vi "NT Process Queued Updates.vi"(9 "Bound Names":string[](array[string]), 11 "handles":cluster{"poller":u32, "topicListener":u32}) -> (3 "Updates":variant[](array[variant]))   [LabVIEW 2025]
uses:
  59b6e50f-ea3d-427c-8cdf-50e68eee575c.vi
  55de3b79-44e1-4c34-8f24-7fb90773489e.vi
  6bfa8e3a-c1d4-42b7-80f0-8f7f4c5a93ba.vi
  b6a8a16d-f334-414e-a614-8fde72f469f3.vi
  <vilib>/Rock Robotics/Network Tables/NT Globals.vi
  <vilib>/Comparison/Equal/Equal Functor/Equal Functor.lvclass
  FRC_NetworkTablesLV.dll
  ntcoreffi.dll
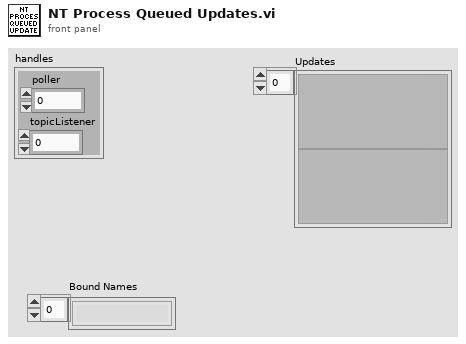
[diagram p1: front panel]
types:
  T1 = cluster{dbl, sgl, i64, string, bool[], dbl[], sgl[], i64[], string[], bool}
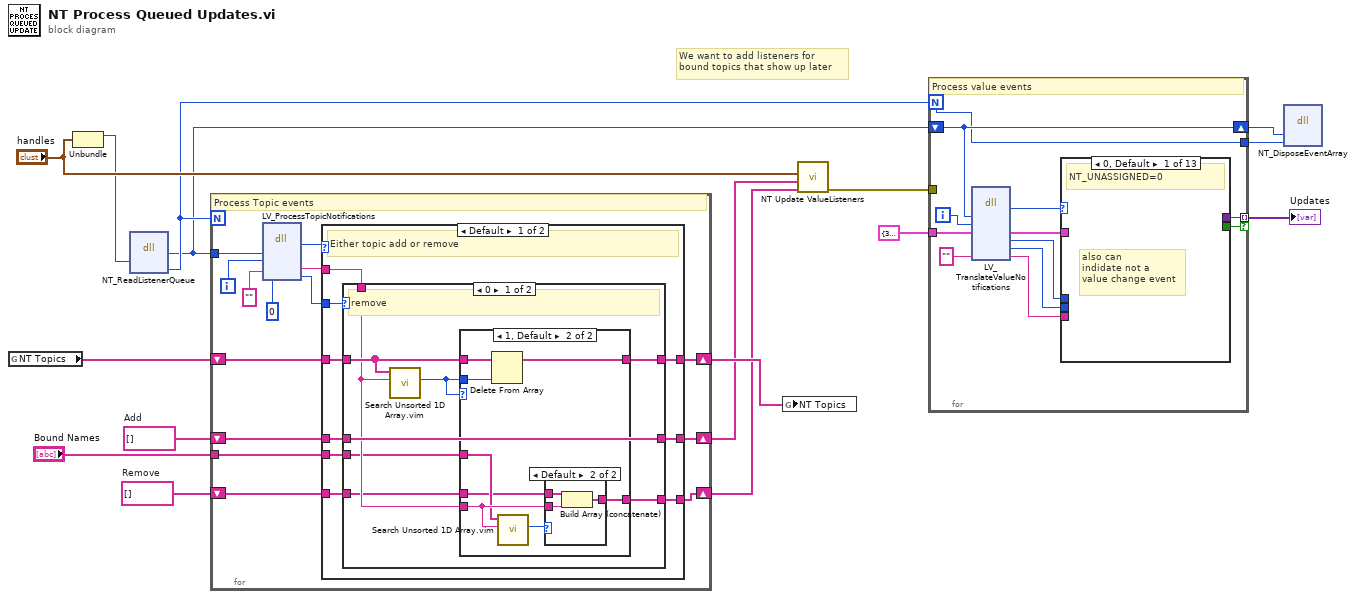
[diagram p0: block diagram]
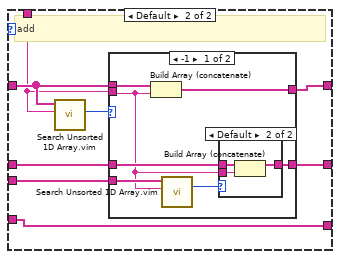
[diagram p4: hidden frame]
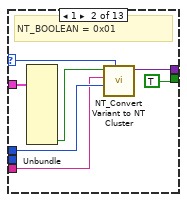
[diagram p8: hidden frame]
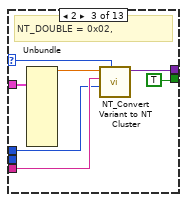
[diagram p9: hidden frame]
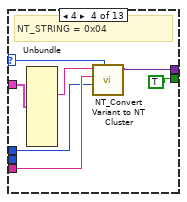
[diagram p10: hidden frame]
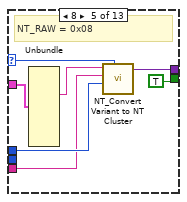
[diagram p11: hidden frame]
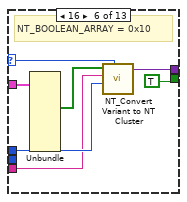
[diagram p12: hidden frame]
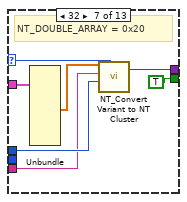
[diagram p13: hidden frame]
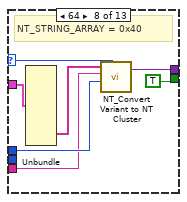
[diagram p14: hidden frame]
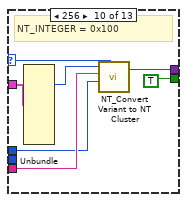
[diagram p16: hidden frame]
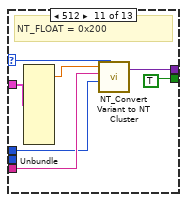
[diagram p17: hidden frame]
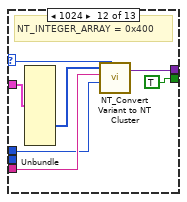
[diagram p18: hidden frame]
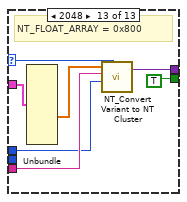
[diagram p19: hidden frame]
diagram:
  w3 = string[] []  # Remove
  w10 = string[] []  # Add
  # "We want to add listeners for\nbound topics that show up later"
  n1 = global read "NT Globals.vi" "NT Topics"() -> (w11:string[])
  n2 = Unbundle("handles") -> ("poller"=w1:u32)  [unwired: 1 out]
  n3 = dll-call lib="ntcoreffi.*" fn="NT_ReadListenerQueue"("poller"=w1) -> ("topicNotif"=w5:u64, "count"=w6:u64)  [unwired: 5 in, 2 out]
  n4 = for {
    N: w6 -> [_]
    tunnel: w5 -> [w30]
    shift-right: [w26] -> w12
    shift-left: w11 -> [w27]
    shift-right: [w24] -> w8
    shift-left: w10 -> [w25]
    tunnel: "Bound Names" -> [w23]
    shift-right: [w17] -> w2
    shift-left: w3 -> [w18]
    i -> [w29]
    # "Process Topic events"
    n5 = dll-call lib="FRC_NetworkTablesLV.*" fn="LV_ProcessTopicNotifications"("topicNotifierArray"=w30, "index"=w29, "name"="", "add"=0) -> ("type"=w21:i32, "name"=w22:string, "add"=w20:i32)  [unwired: 5 in, 2 out]
    n6 = case shown="Default" w21 {
      tunnel: w27 -> [w38 w85]
      tunnel: [w39 w85] -> w26
      tunnel: w25 -> [w37 w84]
      tunnel: [w36 w84] -> w24
      tunnel: w23 -> [w35 _]
      tunnel: w22 -> [w34 _]
      tunnel: w20 -> [w33 _]
      tunnel: w18 -> [w32 w83]
      tunnel: [w31 w83] -> w17
      frame Default {
        # "Either topic add or remove"
        n7 = case shown="0" w33 {
          tunnel: [w46 w69] -> w39
          tunnel: w38 -> [w47 w68]
          tunnel: w37 -> [w44 w66]
          tunnel: [w44 w65] -> w36
          tunnel: w35 -> [w40 w64]
          tunnel: w34 -> [w43 w63]
          tunnel: w32 -> [w42 w62]
          tunnel: [w41 w62] -> w31
          frame 0 {
            # "remove"
            n8 = call "Search Unsorted 1D Array.vim"("element"=w43, "unsorted 1D array"=w47) -> ("index of element"=w45:i32)  [unwired: 9 in]
            n9 = case shown="1, Default" w45 {
              tunnel: w47 -> [w49 w57]
              tunnel: [w49 w56] -> w46
              tunnel: w45 -> [_ w55]
              tunnel: w43 -> [_ w52]
              tunnel: w42 -> [w48 w50]
              tunnel: [w48 w53] -> w41
              tunnel: w40 -> [_ w51]
              frame -1 {
              }
              frame 1, Default {
                n10 = Delete From Array(array=w57, index=w55) -> (array with subset deleted=w56:string[])  [unwired: 1 in, 1 out]
                n11 = call "Search Unsorted 1D Array.vim"("element"=w52, "unsorted 1D array"=w51) -> ("index of element"=w54:i32)  [unwired: 9 in]
                n12 = case shown="Default" w54 {
                  tunnel: w50 -> [w58 w61]
                  tunnel: [w58 w60] -> w53
                  tunnel: w52 -> [_ w59]
                  frame -1 {
                  }
                  frame Default {
                    n13 = Build Array (concatenate)(w61, w59) -> (w60:string[])
                  }
                }
              }
            }
          }
          frame Default {
            # "add"
            n14 = call "Search Unsorted 1D Array.vim"("element"=w63, "unsorted 1D array"=w68) -> ("index of element"=w67:i32)  [unwired: 9 in]
            n15 = case shown="-1" w67 {
              tunnel: w68 -> [w76 w82]
              tunnel: w63 -> [w70 _]
              tunnel: [w75 w82] -> w69
              tunnel: w66 -> [w74 w81]
              tunnel: [w73 w81] -> w65
              tunnel: w64 -> [w71 _]
              frame -1 {
                n16 = Build Array (concatenate)(w76, w70) -> (w75:string[])
                n17 = call "Search Unsorted 1D Array.vim"("element"=w70, "unsorted 1D array"=w71) -> ("index of element"=w72:i32)  [unwired: 9 in]
                n18 = case shown="Default" w72 {
                  tunnel: w74 -> [w77 w80]
                  tunnel: w70 -> [_ w79]
                  tunnel: [w77 w78] -> w73
                  frame -1 {
                  }
                  frame Default {
                    n19 = Build Array (concatenate)(w80, w79) -> (w78:string[])
                  }
                }
              }
              frame Default {
              }
            }
          }
        }
      }
      frame 0 {
        # "Not processed"
      }
    }
  }
  n20 = global write "NT Globals.vi" "NT Topics"(w12) -> ()
  n21 = call <vilib>:"NT Update ValueListeners.vi"("Rm Topics"=w2, "New Topics"=w8, "handles"="handles") -> ("error out"=w4:errorcluster)  [unwired: 8 in]
  n22 = for {
    N: w6 -> [w87]
    tunnel: T1 {3.14, 3.1, 3, "abc", [TRUE], [1.0], [1.0], [1], ["def"], TRUE} -> [w97]
    shift-right: [w95] -> w14
    shift-left: w5 -> [w95]
    tunnel: [w90] -> w15 mode=indexing if=w86
    tunnel: [w87] -> w16
    tunnel: w4 -> [_]
    i -> [w96]
    # "Process value events"
    n23 = dll-call lib="FRC_NetworkTablesLV.*" fn="LV_TranslateValueNotifications"("NTNotifierArray"=w95, "index"=w96, "LVCluster"=w97, "name"="") -> ("type"=w94:i32, "LVCluster"=w93:T1, "time"=w92:i64, "serverTime"=w91:i64, "name"=w88:string)  [unwired: 7 in, 2 out]
    n24 = case shown="0, Default" w94 {
      selector: w94 -> [_ w103 w110 w117 w124 w131 w138 w145 _ w149 w156 w163 w171]
      tunnel: [_ w104 w111 w118 w125 w132 w139 w146 _ w153 w158 w167 w174] -> w90
      tunnel: w93 -> [_ w102 w109 w116 w123 w130 w137 w144 _ w148 w155 w162 w170]
      tunnel: w92 -> [_ w101 w107 w114 w122 w129 w136 w143 _ w150 w159 w164 w168]
      tunnel: w91 -> [_ _ _ _ _ _ _ _ _ _ _ _ _]
      tunnel: w88 -> [_ w100 w108 w115 w121 w128 w135 w142 _ w151 w160 w165 w172]
      tunnel: [_ TRUE TRUE TRUE TRUE TRUE TRUE TRUE _ TRUE TRUE TRUE TRUE] -> w86
      frame 0, Default {
        # "also can\nindidate not a\nvalue change event"
        # "NT_UNASSIGNED=0"
      }
      frame 1 {
        # "NT_BOOLEAN = 0x01"
        n25 = Unbundle(w102) -> (w98:bool)  [unwired: 9 out]
        n26 = call <vilib>:"NT_Convert Variant to NT Cluster.vi"("NT_Type"=w103, "timestamp"=w101, "Name"=w100, "NewVal"=w98) -> ("Value out"=w104:variant)  [unwired: 6 in, 1 out]
      }
      frame 2 {
        # "NT_DOUBLE = 0x02,"
        n27 = Unbundle(w109) -> (w106:dbl)  [unwired: 9 out]
        n28 = call <vilib>:"NT_Convert Variant to NT Cluster.vi"("NT_Type"=w110, "timestamp"=w107, "Name"=w108, "NewVal"=w106) -> ("Value out"=w111:variant)  [unwired: 6 in, 1 out]
      }
      frame 4 {
        # "NT_STRING = 0x04"
        n29 = Unbundle(w116) -> (w112:string)  [unwired: 9 out]
        n30 = call <vilib>:"NT_Convert Variant to NT Cluster.vi"("NT_Type"=w117, "timestamp"=w114, "Name"=w115, "NewVal"=w112) -> ("Value out"=w118:variant)  [unwired: 6 in, 1 out]
      }
      frame 8 {
        # "NT_RAW = 0x08"
        n31 = Unbundle(w123) -> (w119:string)  [unwired: 9 out]
        n32 = call <vilib>:"NT_Convert Variant to NT Cluster.vi"("NT_Type"=w124, "timestamp"=w122, "Name"=w121, "NewVal"=w119) -> ("Value out"=w125:variant)  [unwired: 6 in, 1 out]
      }
      frame 16 {
        # "NT_BOOLEAN_ARRAY = 0x10"
        n33 = Unbundle(w130) -> (w126:bool[])  [unwired: 9 out]
        n34 = call <vilib>:"NT_Convert Variant to NT Cluster.vi"("NT_Type"=w131, "timestamp"=w129, "Name"=w128, "NewVal"=w126) -> ("Value out"=w132:variant)  [unwired: 6 in, 1 out]
      }
      frame 32 {
        # "NT_DOUBLE_ARRAY = 0x20"
        n35 = Unbundle(w137) -> (w133:dbl[])  [unwired: 9 out]
        n36 = call <vilib>:"NT_Convert Variant to NT Cluster.vi"("NT_Type"=w138, "timestamp"=w136, "Name"=w135, "NewVal"=w133) -> ("Value out"=w139:variant)  [unwired: 6 in, 1 out]
      }
      frame 64 {
        # "NT_STRING_ARRAY = 0x40"
        n37 = Unbundle(w144) -> (w140:string[])  [unwired: 9 out]
        n38 = call <vilib>:"NT_Convert Variant to NT Cluster.vi"("NT_Type"=w145, "timestamp"=w143, "Name"=w142, "NewVal"=w140) -> ("Value out"=w146:variant)  [unwired: 6 in, 1 out]
      }
      frame 128 {
        # "NT_RPC = 0x80"
      }
      frame 256 {
        # "NT_INTEGER = 0x100"
        n39 = Unbundle(w148) -> (w147:i64)  [unwired: 9 out]
        n40 = call <vilib>:"NT_Convert Variant to NT Cluster.vi"("NT_Type"=w149, "timestamp"=w150, "Name"=w151, "NewVal"=w147) -> ("Value out"=w153:variant)  [unwired: 6 in, 1 out]
      }
      frame 512 {
        # "NT_FLOAT = 0x200"
        n41 = Unbundle(w155) -> (w154:sgl)  [unwired: 9 out]
        n42 = call <vilib>:"NT_Convert Variant to NT Cluster.vi"("NT_Type"=w156, "timestamp"=w159, "Name"=w160, "NewVal"=w154) -> ("Value out"=w158:variant)  [unwired: 6 in, 1 out]
      }
      frame 1024 {
        # "NT_INTEGER_ARRAY = 0x400"
        n43 = Unbundle(w162) -> (w161:i64[])  [unwired: 9 out]
        n44 = call <vilib>:"NT_Convert Variant to NT Cluster.vi"("NT_Type"=w163, "timestamp"=w164, "Name"=w165, "NewVal"=w161) -> ("Value out"=w167:variant)  [unwired: 6 in, 1 out]
      }
      frame 2048 {
        # "NT_FLOAT_ARRAY = 0x800"
        n45 = Unbundle(w170) -> (w169:sgl[])  [unwired: 9 out]
        n46 = call <vilib>:"NT_Convert Variant to NT Cluster.vi"("NT_Type"=w171, "timestamp"=w168, "Name"=w172, "NewVal"=w169) -> ("Value out"=w174:variant)  [unwired: 6 in, 1 out]
      }
    }
  }
  "Updates" <- w15
  n47 = dll-call lib="ntcoreffi.*" fn="NT_DisposeEventArray"("array"=w14, "count"=w16) -> ()  [unwired: 6 in, 2 out]
